vi "Operational Force Test SAA.vi"(8 "error in (no error)":errorcluster, 10 "Model in":refnum<class "Model.lvclass">, 11 "Test Actuator State in":refnum<class "Test Actuator State.lvclass">) -> (0 "error out":errorcluster, 1 "Pass":bool, 2 "Model out":refnum<class "Model.lvclass">, 3 "Test Actuator State out":refnum<class "Test Actuator State.lvclass">)   [LabVIEW 2016, in "Test Actuator State.lvclass"]
uses:
  Test Actuator State.lvclass
  Model/Model/Model.lvclass
  Typedefs/ActuatorSetPoints.ctl
  <vilib>/Platform/TimedLoop/XDataNode/timing_clust.ctl
  <vilib>/Platform/TimedLoop/XDataNode/nitl_modes.ctl
  <vilib>/Platform/TimedLoop/XDataNode/wakeup.ctl
  Model/Model/Model.lvclass/Model.ctl
  <vilib>/platform/TimedLoop/XDataNode/XDataNode.xnode
  Typedefs/FAMT Typedefs.lvlib
  <vilib>/Platform/TimedLoop/XDataNode/XDNodeRunTimeDep.lvlib
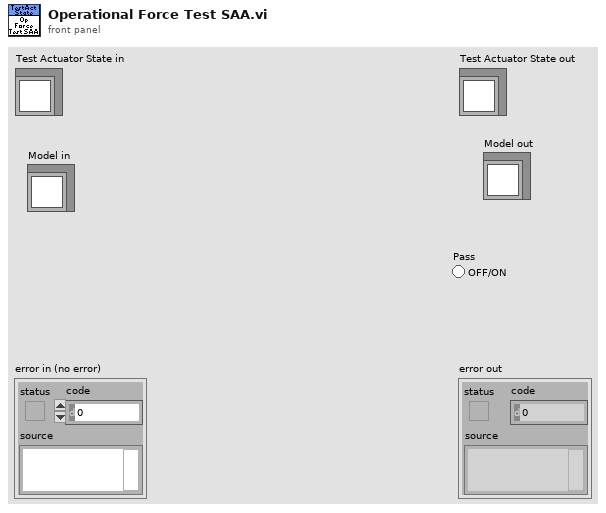
[diagram p1: front panel]
types:
  T1 = typedef "FAMT Typedefs.lvlib/ForcePair.ctl" = cluster{"Axial Force":dbl, "Lateral Force":dbl}
  T2 = typedef "FAMT Typedefs.lvlib/OperationalForceTestSettings.ctl" = cluster{"Max Force Error (N)":dbl, "Max Moment (NM)":dbl, "Process Time (s)":dbl, "Sample Time (s)":dbl}
  T3 = typedef "FAMT Typedefs.lvlib/ActuatorSetPoints.ctl" = cluster{"Axial Force":dbl, "Lateral Force":dbl, "FC1 Force":dbl, "FC2 Force":dbl}
  T4 = typedef "XDNodeRunTimeDep.lvlib/timing_clust.ctl" = cluster{"Expected End [f-1]":u64, "Actual End [f-1]":u64, "Finished Late? [f-1]":bool, "Expected End [i-1]":u64, "Actual End [i-1]":u64, "Finished Late? [i-1]":bool, "Expected Start [i]":u64, "Actual Start [i]":u64, "Expected Start [f]":u64, "Actual Start [f]":u64, "Source Name":string, "Structure Name":string, "Period":i64, "Deadline":i64, "Offset":i64, "Start":i64, "Priority":i32, "Timeout":i32, "Mode":T5, "Wakeup Reason":T6, "Error":errorcluster, "Source Type":string, "Secondary Source Type":string, "Global End Time":u64, "Global Start Time":u64, "Frame Duration":u64, "Iteration Duration":u64, "Assigned CPU":i32, "I/O Scan Engine Mode":u32}
  T5 = typedef "XDNodeRunTimeDep.lvlib/nitl_modes.ctl" = enum32{"No Change", "Process missed periods, maintain original phase", "Discard missed periods, maintain original phase", "Process missed periods, ignore original phase", "Discard missed periods, ignore original phase"}
  T6 = typedef "XDNodeRunTimeDep.lvlib/wakeup.ctl" = enum32{"Normal", "Aborted", "Asynchronous wakeup", "Timing source error", "Timed loop error", "Timeout"}
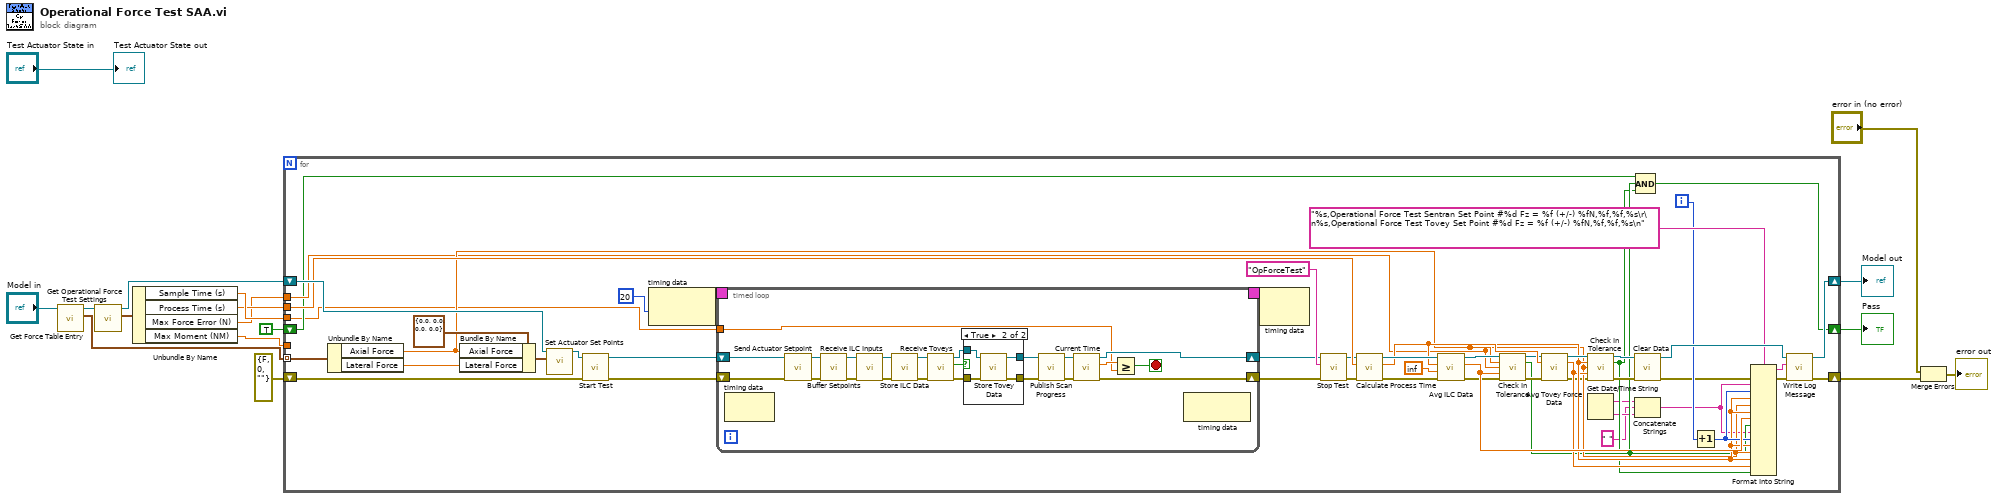
[diagram p0: block diagram]
diagram:
  n1 = call "Get Force Table Entry.vi"("Model in"="Model in") -> ("Entry"=w4:T1[], "Model out"=w7:refnum<class "Model.lvclass">)  [unwired: 8 in, 1 out]
  n2 = call-dynamic "Get Operational Force Test Settings.vi"("Model in"=w7) -> ("Operational Force Test Settings"=w5:T2, "Model out"=w6:refnum<class "Model.lvclass">)  [unwired: 9 in]
  n3 = Unbundle By Name(w5) -> ("Sample Time (s)"=w16:dbl, "Process Time (s)"=w15:dbl, "Max Force Error (N)"=w14:dbl, "Max Moment (NM)"=w9:dbl)
  n4 = for {
    tunnel: w4 -> [w62] mode=indexing
    shift-right: [w66] -> w11
    shift-left: w6 -> [w68]
    tunnel: w16 -> [w26]
    tunnel: w15 -> [w57]
    tunnel: w14 -> [w44]
    shift-right: [w58] -> w10
    shift-left: errorcluster {"status"=FALSE, "code"=0, "source"=""} ("error out") -> [w38]
    tunnel: w9 -> [_]
    shift-right: [w33] -> w1
    shift-left: TRUE -> [w36]
    i -> [w64]
    n5 = Unbundle By Name(w62) -> ("Axial Force"=w48:dbl, "Lateral Force"=w45:dbl)
    n6 = Bundle By Name(cluster=T3 {"Axial Force"=0.0, "Lateral Force"=0.0, "FC1 Force"=0.0, "FC2 Force"=0.0} ("Actuator Set Points"), "Axial Force"=w48, "Lateral Force"=w45) -> (w63:T3)
    n7 = call "Set Actuator Set Points.vi"("Actuator Set Points"=w63, "Model in"=w68) -> ("Model out"=w37:refnum<class "Model.lvclass">)  [unwired: 9 in]
    n8 = call "Start Test.vi"("error in (no error)"=w38, "Model in"=w37) -> ("error out"=w24:errorcluster, "Model out"=w25:refnum<class "Model.lvclass">)  [unwired: 8 in]
    n9 = node-c288(i64 20 ("Period")) -> (w29:T4)
    n10 = timed-loop {
      timing: w29 -> [_]
      timing-out: [_] -> w28
      shift-right: [w73] -> w22
      shift-left: w24 -> [w74]
      shift-right: [w71] -> w23
      shift-left: w25 -> [w72]
      tunnel: w26 -> [w70]
      stop <- w75 stop-if-true
      n11 = node-c288() -> ()  [unwired: 1 in, 1 out]
      n12 = call "Send Actuator Setpoint.vi"("error in (no error)"=w74, "Model in"=w72) -> ("error out"=w90:errorcluster, "Model out"=w88:refnum<class "Model.lvclass">)  [unwired: 8 in]
      n13 = call "Buffer Setpoints.vi"("error in (no error)"=w90, "Model in"=w88) -> ("error out"=w91:errorcluster, "Model out"=w89:refnum<class "Model.lvclass">)  [unwired: 8 in]
      n14 = call "Receive ILC Inputs.vi"("error in (no error)"=w91, "Model in"=w89) -> ("error out"=w77:errorcluster, "Model out"=w76:refnum<class "Model.lvclass">)  [unwired: 8 in]
      n15 = call "Store ILC Data.vi"("error in (no error)"=w77, "Model in"=w76) -> ("error out"=w80:errorcluster, "Model out"=w79:refnum<class "Model.lvclass">)  [unwired: 8 in]
      n16 = call "Receive Toveys.vi"("error in (no error)"=w80, "Model in"=w79) -> ("error out"=w82:errorcluster, "Data Received"=w83:bool, "Model out"=w81:refnum<class "Model.lvclass">)  [unwired: 7 in]
      n17 = case shown="True" w83 {
        tunnel: w81 -> [w93 w97]
        tunnel: w82 -> [w92 w96]
        tunnel: [w92 w95] -> w87
        tunnel: [w93 w94] -> w84
        frame False {
        }
        frame True {
          n18 = call "Store Tovey Data.vi"("error in (no error)"=w96, "Model in"=w97) -> ("error out"=w95:errorcluster, "Model out"=w94:refnum<class "Model.lvclass">)  [unwired: 8 in]
        }
      }
      n19 = call "Publish Scan Progress.vi"("error in (no error)"=w87, "Model in"=w84) -> ("error out"=w86:errorcluster, "Model out"=w85:refnum<class "Model.lvclass">)  [unwired: 8 in]
      n20 = call "Current Time.vi"("error in (no error)"=w86, "Model in"=w85) -> ("error out"=w73:errorcluster, "Time"=w78:dbl, "Model out"=w71:refnum<class "Model.lvclass">)  [unwired: 7 in]
      n21 = Greater Or Equal?(x=w78, y=w70) -> (x >= y?=w75:bool)
      n22 = node-c288() -> ()  [unwired: 1 in, 1 out]
    }
    n23 = node-c288(w28) -> ()  [unwired: 1 out]
    n24 = call "Stop Test.vi"("error in (no error)"=w22, "Test"="OpForceTest", "Model in"=w23) -> ("error out"=w31:errorcluster, "Model out"=w32:refnum<class "Model.lvclass">)  [unwired: 7 in]
    n25 = call "Calculate Process Time.vi"("error in (no error)"=w31, "Seconds"=w57, "Model in"=w32) -> ("error out"=w55:errorcluster, "Time"=w54:dbl, "Model out"=w56:refnum<class "Model.lvclass">)  [unwired: 6 in]
    n26 = call "Avg ILC Data.vi"("error in (no error)"=w55, "Before This Time"=inf, "After This Time"=w54, "Model in"=w56) -> ("error out"=w51:errorcluster, "Fz"=w52:dbl, "Model out"=w53:refnum<class "Model.lvclass">)  [unwired: 4 in, 1 out]
    n27 = call "Check In Tolerance.vi"("Model in"=w53, "Expected"=w48, "Tolerance"=w44, "Actual"=w52, "error in (no error)"=w51) -> ("Model out"=w41:refnum<class "Model.lvclass">, "Pass"=w35:bool, "error out"=w40:errorcluster)  [unwired: 8 in]
    n28 = call "Avg Tovey Force Data.vi"("Model in"=w41, "After This Time"=w54, "error in (no error)"=w40) -> ("Model out"=w49:refnum<class "Model.lvclass">, "Fz"=w47:dbl, "error out"=w43:errorcluster)  [unwired: 8 in, 2 out]
    n29 = call "Check In Tolerance.vi"("Model in"=w49, "Expected"=w48, "Tolerance"=w44, "Actual"=w47, "error in (no error)"=w43) -> ("Model out"=w46:refnum<class "Model.lvclass">, "Pass"=w34:bool, "error out"=w42:errorcluster)  [unwired: 8 in]
    n30 = Get Date/Time String() -> (date string=w21:string, time string=w20:string)  [unwired: 3 in]
    n31 = call "Clear Data.vi"("error in (no error)"=w42, "Model in"=w46) -> ("error out"=w60:errorcluster, "Model out"=w67:refnum<class "Model.lvclass">)  [unwired: 8 in]
    n32 = Concatenate Strings(w21, " " ("string"), w20) -> (w18:string)
    n33 = Compound Arithmetic op=AND(w36, w35, w34) -> (w33:bool)
    n34 = Increment(x=w64) -> (x+1=w50:i32)
    n35 = Format Into String(format string="%s,Operational Force Test Sentran Set Point #%d Fz = %f (+/-) %fN,%f,%f,%s\r\n%s,Operational Force Test Tovey Set Point #%d Fz = %f (+/-) %fN,%f,%f,%s\n", error in=w60, w18, w50, w48, w44, w48, w52, w35, w18, w50, w48, w44, w48, w47, w34) -> (resulting string=w61:string, error out=w59:errorcluster)  [unwired: 1 in]
    n36 = call "Write Log Message.vi"("error in (no error)"=w59, "Message"=w61, "Model in"=w67) -> ("error out"=w58:errorcluster, "Model out"=w66:refnum<class "Model.lvclass">)  [unwired: 7 in]
  }
  "Model out" <- w11
  "Pass" <- w1
  n37 = Merge Errors("error in (no error)", w10) -> (→"error out":errorcluster)
  "Test Actuator State out" <- "Test Actuator State in"
